vi "SV name extractor.vi"(11 "Refnum in":refnum<k21>) -> (3 "String":string)   [LabVIEW 2026, in "TALOS.lvlib"]
uses:
  TALOS.lvlib
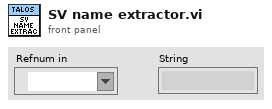
[diagram p1: front panel]
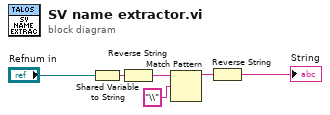
[diagram p0: block diagram]
diagram:
  n1 = Shared Variable to String(1:"Refnum in") -> (0:w4:string)
  n2 = Reverse String(1:w4) -> (0:w3:string)
  n3 = Match Pattern(string=w3, regular expression="\\") -> (before substring=w2:string)  [unwired: 1 in, 3 out]
  n4 = Reverse String(1:w2) -> (0:→"String":string)
